vi "Write CellData.vi"(8 "error in":errorcluster, 10 "CellData":refnum<class "PAS Cell Data.lvclass">[](array[class]), 11 "PAS Data in":refnum<class "PAS Data.lvclass">) -> (0 "error out":errorcluster, 3 "PAS Data out":refnum<class "PAS Data.lvclass">)   [LabVIEW 2018, in "PAS Library.lvlib" / "PAS Data.lvclass"]
uses:
  PAS Data.lvclass
  Cell/PAS Cell Data.lvclass
  PAS Data.lvclass/PAS Data.ctl
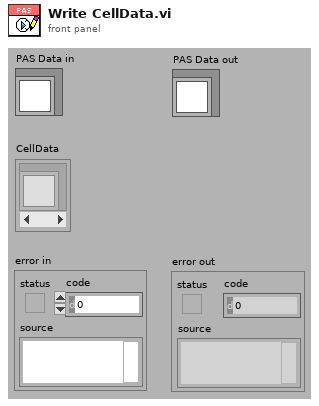
[diagram p1: front panel]
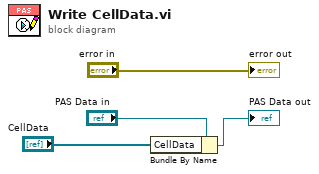
[diagram p0: block diagram]
diagram:
  n1 = Bundle By Name(cluster="PAS Data in", "CellData"="CellData") -> (→"PAS Data out":refnum<class "PAS Data.lvclass">)
  "error out" <- "error in"
